vi "Testing I16 to FXP18 conversions.vi"() -> ()   [LabVIEW 2015]
uses:
  DDC_7976R_v1.lvlib
  <vilib>/Analysis/NI_AALBase.lvlib
panel:
  in  "element":dbl format="%#_13g"
  out "appended array":dbl[][](graph)
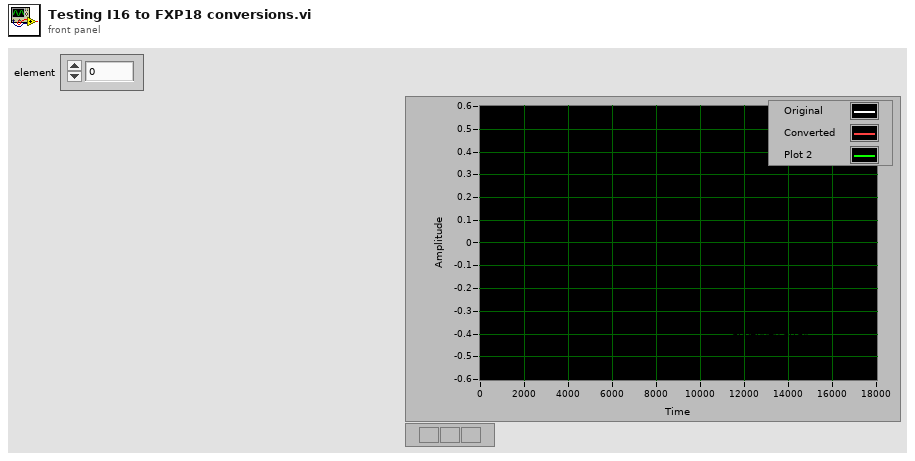
[diagram p1: front panel]
types:
  T1 = typedef "niInstr DSP v1 Shared.lvlib/IQ Data.ctl" = cluster{"I":fxp<+/-,18,1>, "Q":fxp<+/-,18,1>, "overflow":bool}
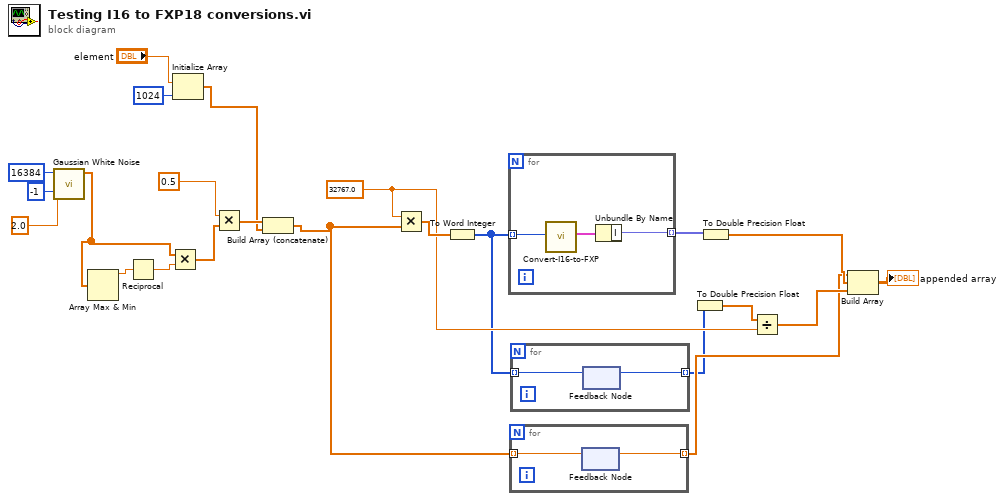
[diagram p0: block diagram]
diagram:
  w11 = 32767.0
  n1 = call <vilib>:"Gaussian White Noise.vi"("seed"=-1, "standard deviation"=2.0, "samples"=16384) -> ("Gaussian noise pattern"=w18:dbl[])  [unwired: 7 in, 1 out]
  n2 = Array Max & Min(array=w18) -> (max value=w19:dbl)  [unwired: 3 out]
  n3 = Reciprocal(x=w19) -> (1/x=w17:dbl)
  n4 = Multiply(x=w18, y=w17) -> (x*y=w16:dbl[])
  n5 = Initialize Array("element", 1024 ("dimension size")) -> (w6:dbl[])
  n6 = Multiply(x=0.5, y=w16) -> (x*y=w7:dbl[])
  n7 = Build Array (concatenate)(w7, w6) -> (w4:dbl[])
  n8 = Multiply(x=w11, y=w4) -> (x*y=w15:dbl[])
  n9 = To Word Integer(number=w15) -> (16bit integer=w2:i16[])
  n10 = for {
    tunnel: w2 -> [w26] mode=indexing
    tunnel: [w24] -> w14 mode=indexing
    n11 = call "Convert-I16-to-FXP.vi"("I16 in"=w26) -> ("data out"=w25:T1)  [unwired: 6 in]
    n12 = Unbundle By Name(w25) -> ("I"=w24:fxp<+/-,18,1>)
  }
  n13 = for {
    tunnel: w4 -> [w28] mode=indexing
    tunnel: [w27] -> w3 mode=indexing
    n14 = feedback #1() -> (w27:dbl)  [unwired: 1 in]
    n15 = feedback-in #1(w28) -> ()
  }
  n16 = for {
    tunnel: w2 -> [w30] mode=indexing
    tunnel: [w29] -> w1 mode=indexing
    n17 = feedback #2() -> (w29:i16)  [unwired: 1 in]
    n18 = feedback-in #2(w30) -> ()
  }
  n19 = To Double Precision Float(number=w1) -> (double precision float=w12:dbl[])
  n20 = To Double Precision Float(number=w14) -> (double precision float=w5:dbl[])
  n21 = Divide(x=w12, y=w11) -> (x/y=w10:dbl[])
  n22 = Build Array(w3, w5, w10) -> (→"appended array":dbl[][])
